vi "Excitation_Gen.vi"(4 "Current Frequency Index":i32, 5 "Current Sample":i32, 6 "Samples Before Frequency Change":i32[](array[numeric]), 7 "Excitation Frequencies":dbl[](array[numeric]), 8 "Excitation Specs":T1) -> (0 "In Frequency Sinusoids":cluster{"cos(wt)":dbl, " sin(wt)":dbl}, 1 "Excitation Sinusoid":dbl, 2 "Current Frequency":dbl, 3 "New Frequency Index":i32)   [LabVIEW 2020, in "DynamicSignalAnalyzer.lvlib"]
doc: "Outputs a point by point swept sine wave, the frequency of the sine wave for the current point, and the index of the frequency within the list excitation frequencies that this function will generate the sine wave at for the next point.\n\nInputs:\n\n- Current Frequency Index: The index of the current frequency being used to generate the current sine wave within the input excitation frequencies.\n\n- Excitiation Frequencies: A list of spaced out frequencies to generate a swept sine wave (multiple sine waves with different frequencies).\n\n- Excitation Specs:\n - Used: Amplitude, Sampling Time, & Offset\n - Not: Initial Frequency, Final Frequency, Frequency Units, Number of Frequencies\n\n- Samples Before Frequency Change: A list of the indices of the last sample taken at a particular frequency before the frequency changes. The following sample, the excitaton frequency changes. \n\n- Current Sample: The current sample being generated to excite the system\n\nOutputs:\n\n- New Frequency Index: The index of the frequency within the list of excitation frequencies that this function will generate the sine wave at on it's next iteration. \n\n- Current Frequency: The frequency of the sine wave generate for the current sample.\n\n- Sinusoid Excitation: A point by point (thus this output is a single float number, not a list) swept sine wave to excite the system with. \n\n- In Frequency Sinusoids: A point by point (thus this output is a single float number, not a list) sine and cosine wave at the frequencies of the swept sine wave without the swept sine wave's DC offset to demodulate the system's frequency response to pull out the phase and magnitude."
uses:
  DynamicSignalAnalyzer.lvlib
  <vilib>/ptbypt/NI_PtbyPt.lvlib
panel:
  # "Excitation_Generator"
  # "Current Data"
  # "Excitation Properties"
  # "In Frequency Sinusoids"
  # "Excitation Frequencies"
  # "Frequency\nUnits"
  # "[Hz]"
  # "Excitation Magnitude"
  # "[rad/s]"
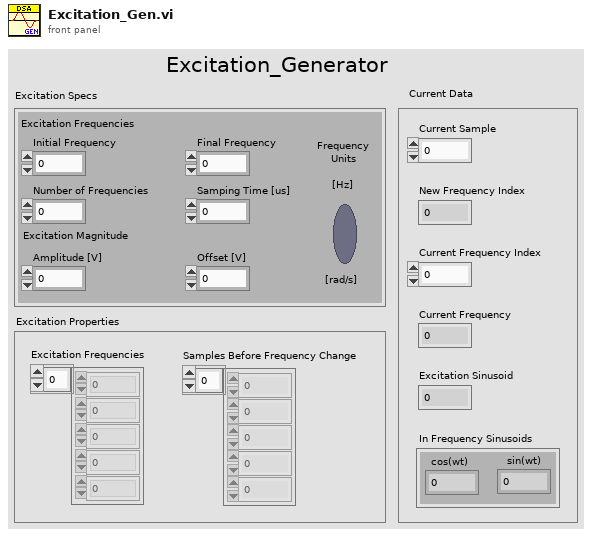
[diagram p1: front panel]
types:
  T1 = cluster{"Initial Frequency":dbl, "Final Frequency":dbl, "Number of Frequencies":i16, "Samping Time [us]":dbl, "Amplitude [V]":dbl, "Offset [V]":dbl, "Freq Unit":bool}
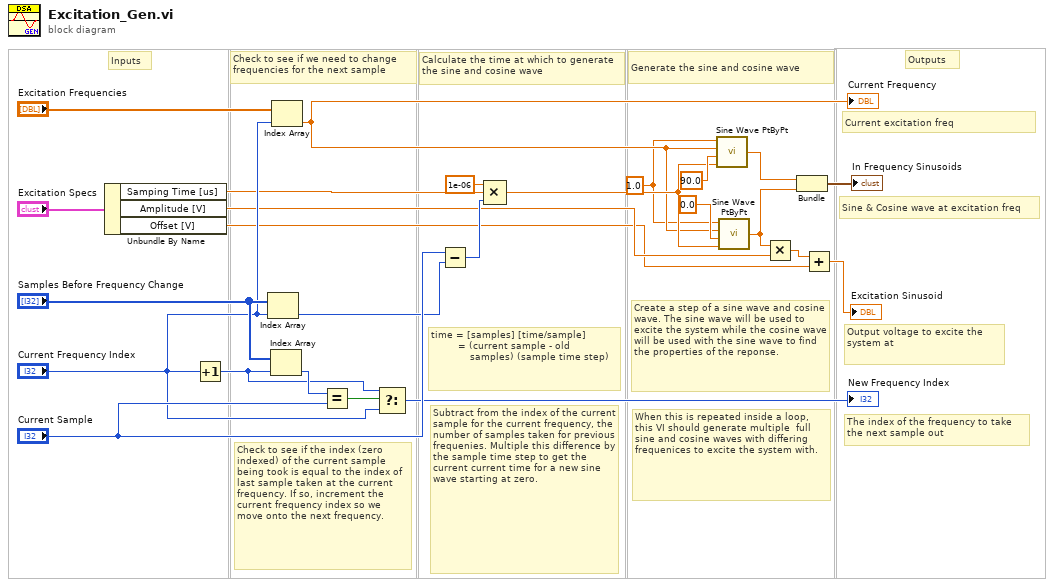
[diagram p0: block diagram]
diagram:
  w9 = 1.0
  # "Current excitation freq"
  # "Sine & Cosine wave at excitation freq"
  # "Output voltage to excite the system at"
  # "The index of the frequency to take the next sample out"
  # "Generate the sine and cosine wave"
  # "Calculate the time at which to generate the sine and cosine wave"
  # "Check to see if we need to change frequencies for the next sample"
  # "Outputs"
  # "When this is repeated inside a loop, this VI should generate multiple  full sine and cosine waves with differing frequenices to excite the system with."
  # "Create a step of a sine wave and cosine wave. The sine wave will be used to excite the system while the cosine wave will be used with the sine wave to find the properties of the reponse."
  # "time = [samples] [time/sample]\n         = (current sample - old               \n             samples) (sample time step)"
  # "Subtract from the index of the current sample for the current frequency, the number of samples taken for previous frequenies. Multiple this difference by the sample time step to get the current current time for a new sine wave starting at zero."
  # "Check to see if the index (zero indexed) of the current sample being took is equal to the index of last sample taken at the current frequency. If so, increment the current frequency index so we move onto the next frequency."
  # "Inputs"
  n1 = Unbundle By Name("Excitation Specs") -> ("Samping Time [us]"=w6:dbl, "Amplitude [V]"=w5:dbl, "Offset [V]"=w4:dbl)
  n2 = Increment(x="Current Frequency Index") -> (x+1=w22:i32)
  n3 = Index Array(array="Samples Before Frequency Change", index="Current Frequency Index") -> (element=w20:i32)
  n4 = Index Array(array="Samples Before Frequency Change", index=w22) -> (element=w23:i32)
  n5 = Index Array(array="Excitation Frequencies", index="Current Frequency Index") -> (element=w12:dbl)
  "Current Frequency" <- w12
  n6 = Equal?(x=w23, y="Current Sample") -> (x = y?=w3:bool)
  n7 = Select(t=w22, s=w3, f="Current Frequency Index") -> (s? t:f=→"New Frequency Index":i32)
  n8 = Subtract(x="Current Sample", y=w20) -> (x-y=w18:i32)
  n9 = Compound Arithmetic op=MULTIPLY(1e-06 ("value"), w6, w18) -> (w13:dbl)
  n10 = call <vilib>:"Sine Wave PtByPt.vi"("time"=w13, "phase"=90.0, "frequency"=w12, "amplitude"=w9) -> ("sine wave"=w10:dbl)
  n11 = call <vilib>:"Sine Wave PtByPt.vi"("time"=w13, "phase"=0.0, "frequency"=w12, "amplitude"=w9) -> ("sine wave"=w8:dbl)
  n12 = Multiply(x=w8, y=w5) -> (x*y=w7:dbl)
  n13 = Bundle("sine wave"=w10, "sine wave"=w8) -> (→"In Frequency Sinusoids":cluster{"sine wave":dbl, "sine wave":dbl})  [unwired: 1 in]
  n14 = Add(x=w7, y=w4) -> (x+y=→"Excitation Sinusoid":dbl)
